vi "AI RTM Enable Disable Dependency.vi"(8 "error in (no error)":errorcluster, 10 "Menu hierarchy in":string[](array[string]), 11 "Node Ref":T2 format="%.0x") -> (0 "error out":errorcluster, 2 "Menu hierarchy out":string[](array[string]), 3 "Action":T1)   [LabVIEW 2013]
uses:
  <vilib>/K2Labs/HiLab API/Custom Device API/Controls/Custom Device Item Reference.ctl
  <vilib>/K2Labs/HiLab API/Custom Device API/Controls/Custom Device RTM Dependency.ctl
  <vilib>/K2Labs/HiLab API/Custom Device API/Configuration/Item Properties/Get Item Property/Get Item Property.xnode
  <vilib>/K2Labs/HiLab API/Custom Device API/Custom Device API Library.lvlib
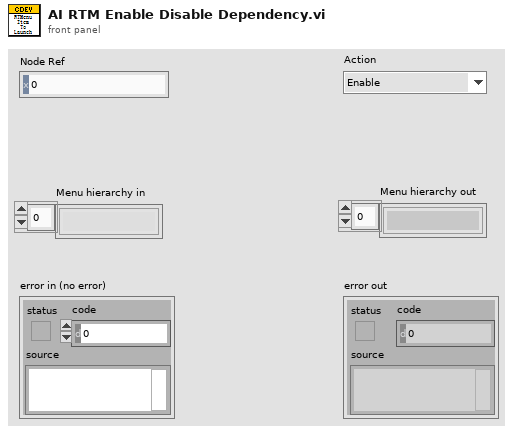
[diagram p1: front panel]
types:
  T1 = typedef "Custom Device API Library.lvlib/Custom Device RTM Dependency.ctl" = enum16{"Enable", "Disable", "Hide"}
  T2 = typedef "Custom Device API Library.lvlib/Custom Device Item Reference.ctl" = u64
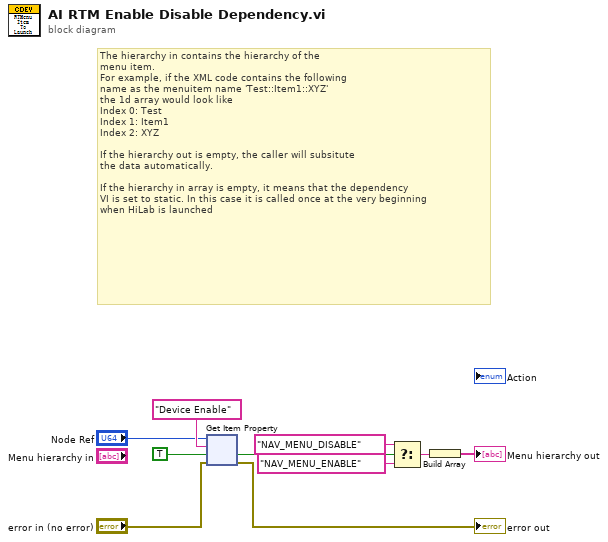
[diagram p0: block diagram]
diagram:
  # "The hierarchy in contains the hierarchy of the\nmenu item.\nFor example, if the XML code contains the following\nname as the menuitem name 'Test::Item1::XYZ'\nthe 1d array would look like\nIndex 0: Test\nIndex 1: Item1\nIndex 2: XYZ\n\nIf the hierarchy out is empty, the caller will subsitute\nthe data automatically.\n\nIf the hierarchy in array is empty, it means that the dependency\nVI is set to static. In this case it is called once at the very beginning\nwhen HiLab is launched"
  n1 = xnode "Get Item Property"("Item Ref in"="Node Ref", "Property Name"="Device Enable", "Default Value"=TRUE, "error in (no error)"="error in (no error)") -> ("Value"=w1:bool, "error out"=→"error out":errorcluster)  [unwired: 2 out]
  n2 = Select(t="NAV_MENU_DISABLE" ("y"), s=w1, f="NAV_MENU_ENABLE") -> (s? t:f=w8:string)
  n3 = Build Array(w8) -> (→"Menu hierarchy out":string[])
